vi "Bump test M-11.vi"() -> ()   [LabVIEW 2018]
doc: "This VI is an example of using the PID VI for a PWM application. For a real application all that is needed is the PID VI and the Output to PWM Logic. Together these can be put in the while loop of a real application.\n\nThis example has defaults tuned to the plant."
uses:
  <vilib>/ptbypt/NI_PtbyPt.lvlib
panel:
  out "Waveform Chart 2":dbl(graph)
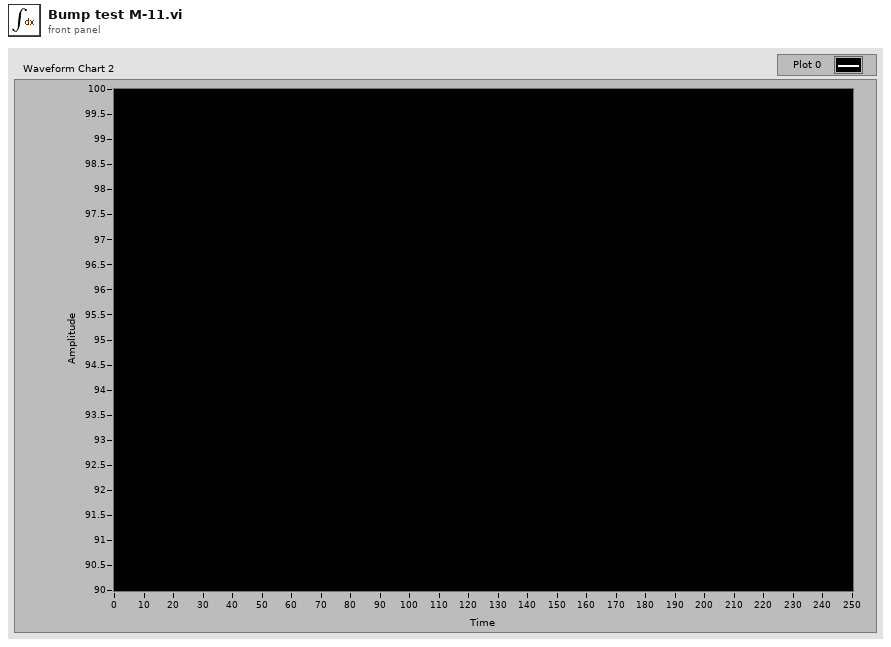
[diagram p1: front panel]
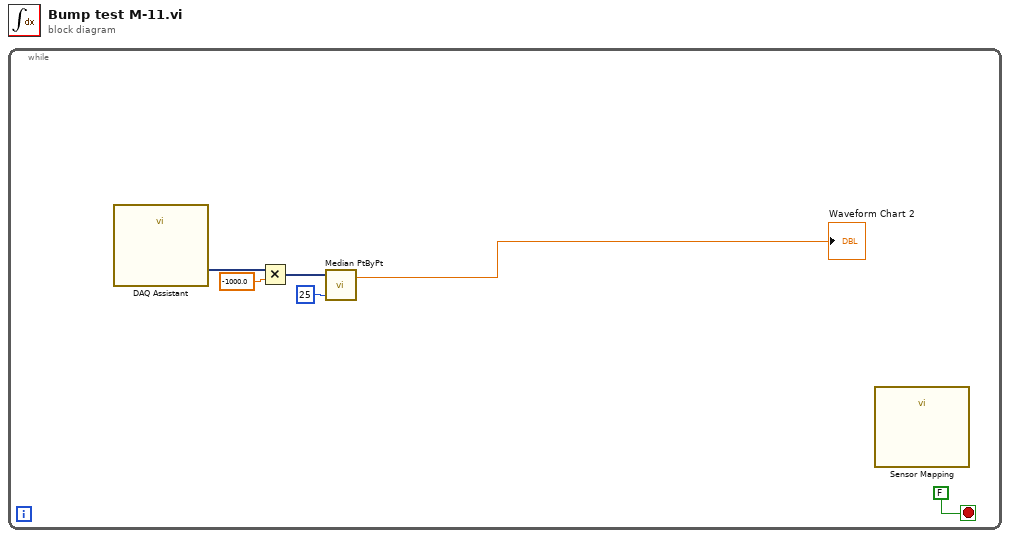
[diagram p0: block diagram]
diagram:
  n1 = while {
    stop <- FALSE stop-if-true
    n2 = call "DAQ Assistant"() -> ("data"=w6:dynamicdata)  [unwired: 17 in, 2 out]
    n3 = Multiply(x=w6, y=-1000.0) -> (x*y=w4:dynamicdata)
    n4 = call <vilib>:"Median PtByPt.vi"("sample length"=25, "x"=w4) -> ("median"=→"Waveform Chart 2":dbl)  [unwired: 2 in, 1 out]
    n5 = call "Sensor Mapping"() -> ()  [unwired: 10 in, 2 out]
  }
